vi "SetBounds.vi"(8 "error in (no error)":errorcluster, 10 "bounds":cluster{"width":u32, "height":u32}, 11 "overlay in":refnum<class "overlay.lvclass">) -> (0 "error out":errorcluster, 3 "overlay out":refnum<class "overlay.lvclass">)   [LabVIEW 2009, in "overlay.lvclass"]
uses:
  overlay.lvclass
  overlay.lvclass/overlay.ctl
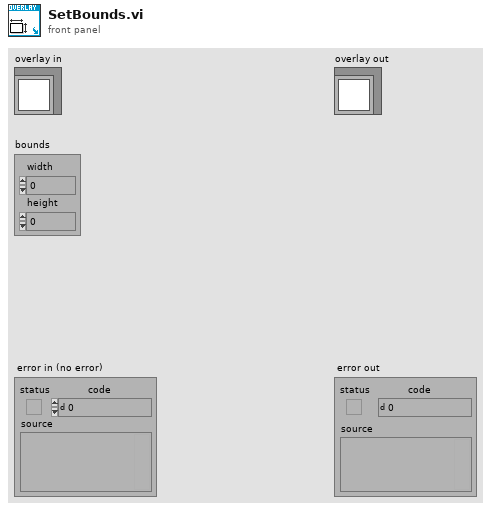
[diagram p1: front panel]
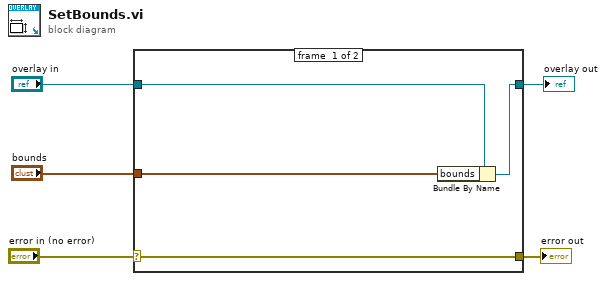
[diagram p0: block diagram]
diagram:
  n1 = case shown="No Error" "error in (no error)" {
    selector: "error in (no error)" -> [w9 w10]
    tunnel: [w9 w10] -> w2
    tunnel: [w7 w11] -> w4
    tunnel: "overlay in" -> [w8 w11]
    tunnel: "bounds" -> [w6 _]
    frame #0 {
      n2 = Bundle By Name(cluster=w8, "bounds"=w6) -> (w7:refnum<class "overlay.lvclass">)
    }
    frame #1 {
    }
  }
  "error out" <- w2
  "overlay out" <- w4
